vi "APTmotorClose.vi"(8 "error in (no error)":errorcluster, 11 "reference in":refnum<k7>[](array[refnum])) -> (0 "error out":errorcluster)   [LabVIEW 2015]
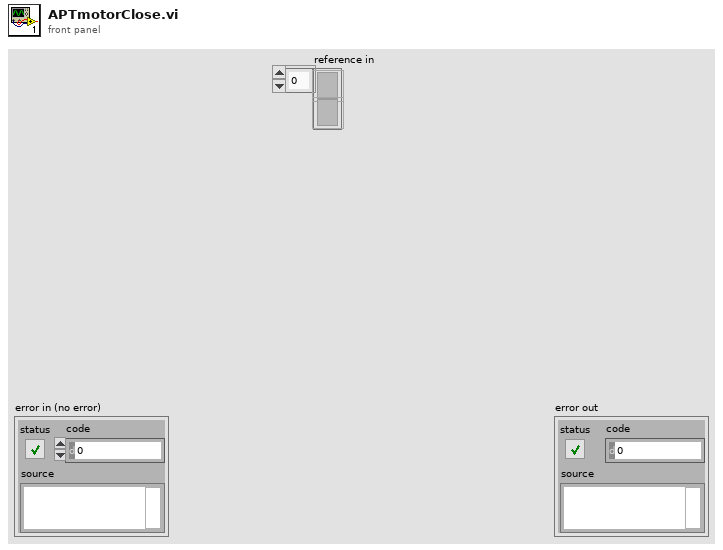
[diagram p1: front panel]
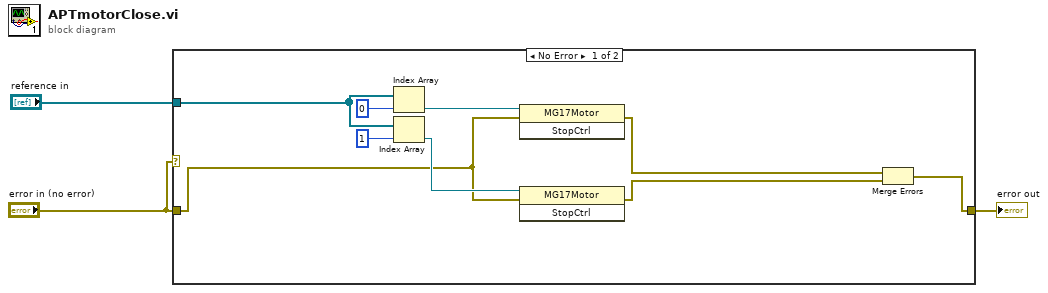
[diagram p0: block diagram]
diagram:
  n1 = case shown="No Error" "error in (no error)" {
    tunnel: [w7 w13] -> w3
    tunnel: "error in (no error)" -> [w8 w13]
    tunnel: "reference in" -> [w6 _]
    frame No Error {
      n2 = Index Array(array=w6, index=0) -> (element=w11:refnum<k7>)
      n3 = Index Array(array=w6, index=1) -> (element=w9:refnum<k7>)
      n4 = invoke class="MG17Motor" method="StopCtrl"(reference=w11, error in=w8) -> (error out=w5:errorcluster)  [unwired: 1 in, 2 out]
      n5 = invoke class="MG17Motor" method="StopCtrl"(reference=w9, error in=w8) -> (error out=w4:errorcluster)  [unwired: 1 in, 2 out]
      n6 = Merge Errors(w5, w4) -> (w7:errorcluster)
    }
    frame Error {
    }
  }
  "error out" <- w3
